vi "Decimate DFD (Fs).vi"(8 "error in (no error)":errorcluster, 10 "output fs[Hz]":dbl=6500.0 format="%#_13g", 11 "Waveforms in":waveform(dbl)[](array[waveform])) -> (0 "error out":errorcluster, 3 "waveforms out":waveform(dbl)[](array[waveform]))   [LabVIEW 2019, in "Instrument.Lockin.lvlib" / "Instrument.DAQ.lvclass"]
uses:
  Instrument.DAQ.lvclass
  <vilib>/Utility/error.llb/Clear Errors.vi
  <vilib>/Analysis/2dsp.llb/Decimate (single shot).vi
  <vilib>/Analysis/2dsp.llb/Decimate (single shot, DBL).vi
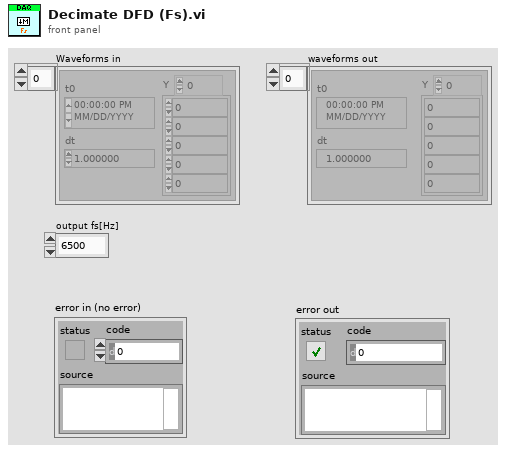
[diagram p1: front panel]
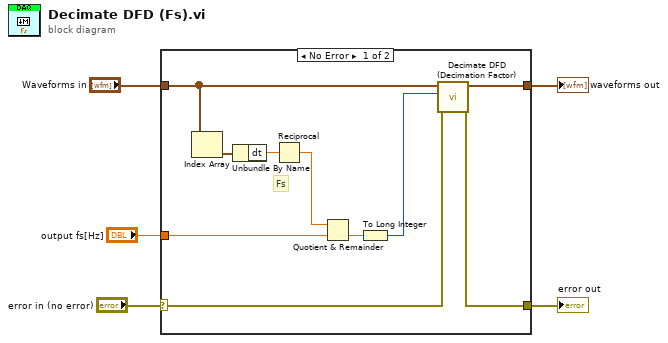
[diagram p0: block diagram]
diagram:
  n1 = case shown="No Error" "error in (no error)" {
    selector: "error in (no error)" -> [w8 w17]
    tunnel: "output fs[Hz]" -> [w11 _]
    tunnel: "Waveforms in" -> [w10 w16]
    tunnel: [w7 w17] -> w2
    tunnel: [w9 w16] -> w1
    frame No Error {
      # "Fs"
      n2 = Index Array(array=w10) -> (element=w14:waveform(dbl))  [unwired: 1 in]
      n3 = Unbundle By Name(w14) -> ("dt"=w13:dbl)
      n4 = Reciprocal(x=w13) -> (1/x=w12:dbl)
      n5 = Quotient & Remainder(x=w12, y=w11) -> (floor(x/y)=w15:dbl)  [unwired: 1 out]
      n6 = To Long Integer(number=w15) -> (32bit integer=w6:i32)
      n7 = call "Decimate DFD (Decimation Factor).vi"("error in (no error)"=w8, "Decimation Factor"=w6, "Waveforms in"=w10) -> ("error out"=w7:errorcluster, "waveforms out"=w9:waveform(dbl)[])  [unwired: 7 in]
    }
    frame Error {
    }
  }
  "waveforms out" <- w1
  "error out" <- w2
